vi "Send simulated.vi"(8 "error in (no error)":errorcluster, 10 "Channel":enum16{"2", "1"}(ring), 11 "Simulated Device in":refnum<class "Simulated Device.lvclass">) -> (0 "error out":errorcluster, 2 "Response":i32, 3 "Simulated Device out":refnum<class "Simulated Device.lvclass">)   [LabVIEW 2020, in "Simulated Device.lvclass"]
uses:
  Simulated Device.lvclass
  da403052-b189-4cca-8cb5-0a9d17cf4de7.vi
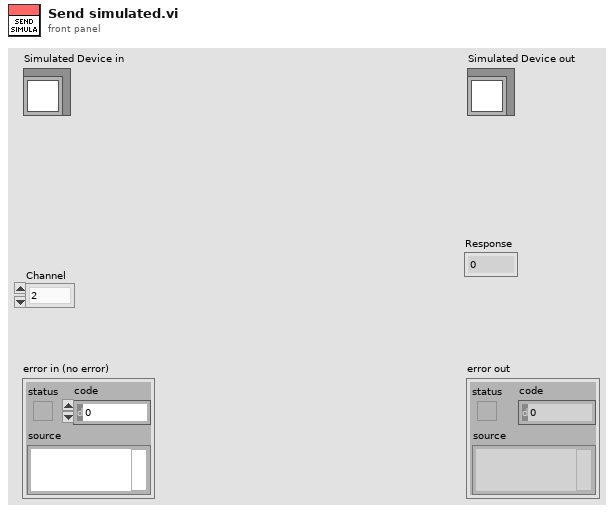
[diagram p1: front panel]
types:
  T1 = enum16{"Write", "Read", "Config", "Reset", "Close"}
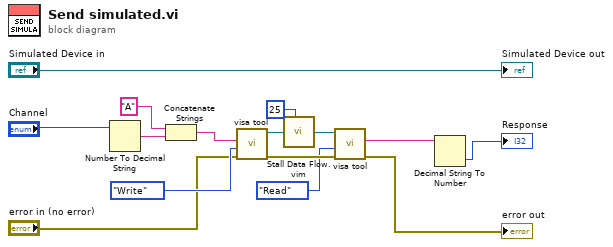
[diagram p0: block diagram]
diagram:
  n1 = Number To Decimal String(number="Channel") -> (decimal integer string=w14:string)  [unwired: 1 in]
  n2 = Concatenate Strings("A" ("string"), w14) -> (w13:string)
  n3 = call "visa tool.vi"("error in (no error)"="error in (no error)", "Opciones"=T1."Write", "Write"=w13) -> ("error out"=w9:errorcluster, "VISA com port 2"=w11:refnum<visa-resource-name>)  [unwired: 6 in, 1 out]
  n4 = call "Stall Data Flow.vim"("value in"=w11, "milliseconds to wait"=u32 25) -> ("value out"=w10:refnum<visa-resource-name>)  [unwired: 1 out]
  n5 = call "visa tool.vi"("error in (no error)"=w9, "Opciones"=T1."Read", "VISA com port"=w10) -> ("error out"=→"error out":errorcluster, "Read"=w8:string)  [unwired: 6 in, 1 out]
  n6 = Decimal String To Number(string=w8) -> (number=→"Response":i32)  [unwired: 2 in, 1 out]
  "Simulated Device out" <- "Simulated Device in"
